vi "get array from image file.vi"(8 "error in (no error)":errorcluster, 10 "File Path":path, 11 "Autofocus in":refnum<class "Autofocus.lvclass">) -> (0 "error out":errorcluster, 3 "Autofocus out":refnum<class "Autofocus.lvclass">)   [LabVIEW 2012, in "Autofocus.lvclass"]
uses:
  Autofocus.lvclass
  Autofocus.lvclass/Autofocus.ctl
panel:
  out "Image Source":T1(plugin-control)
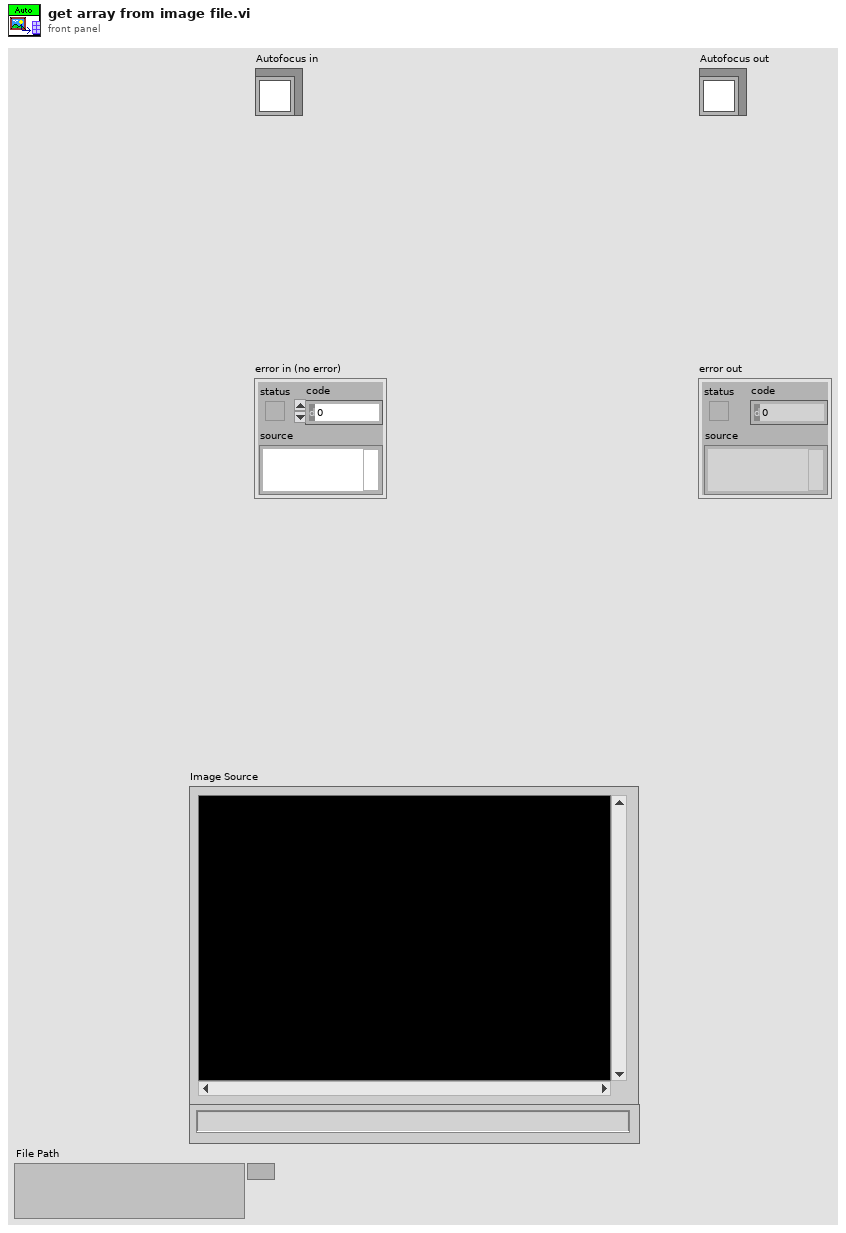
[diagram p1: front panel]
types:
  T1 = typedef "IMAQ Image.ctl" = refnum<image>
  T2 = typedef "Image Type" = u32
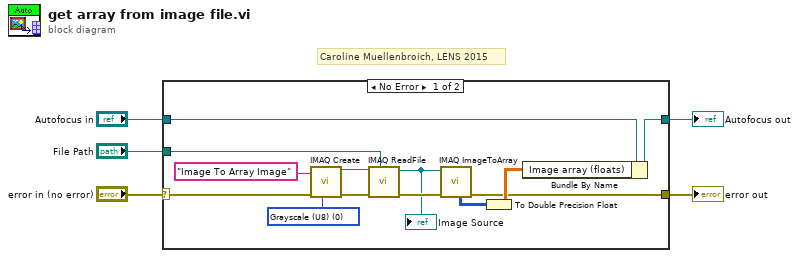
[diagram p0: block diagram]
diagram:
  # "Caroline Muellenbroich, LENS 2015"
  n1 = case shown="No Error" "error in (no error)" {
    selector: "error in (no error)" -> [w10 w20]
    tunnel: [w9 w20] -> w4
    tunnel: [w12 w19] -> w2
    tunnel: "Autofocus in" -> [w13 w19]
    tunnel: "File Path" -> [w7 _]
    frame No Error {
      w15 = T2 0 items=["Grayscale (U8)", "Grayscale (I16)", "Grayscale (SGL)", "Complex (CSG)", "RGB (U32)", "HSL (U32)", "RGB (U64)", "Grayscale (U16)"] ("Image Type")
      n2 = call "IMAQ Create"("Image Name"="Image To Array Image", "Image Type"=w15, "error in (no error)"=w10) -> ("New Image"=w16:T1, "error out"=w17:errorcluster)  [unwired: 2 in]
      n3 = call "IMAQ ReadFile"("File Path"=w7, "error in (no error)"=w17, "Image"=w16) -> ("error out"=w14:errorcluster, "Image Out"=w8:T1)  [unwired: 4 in, 3 out]
      "Image Source" <- w8
      n4 = call "IMAQ ImageToArray"("error in (no error)"=w14, "Image"=w8) -> ("Image Pixels (U16)"=w6:u16[][], "error out"=w9:errorcluster)  [unwired: 2 in, 3 out]
      n5 = To Double Precision Float(number=w6) -> (double precision float=w11:dbl[][])
      n6 = Bundle By Name(cluster=w13, "Image array (floats)"=w11) -> (w12:refnum<class "Autofocus.lvclass">)
    }
    frame Error {
    }
  }
  "error out" <- w4
  "Autofocus out" <- w2
